vi "找螺丝刀方向-两头.vi"(8 "螺丝刀重心":cluster{"X":sgl, "Y":sgl} {"Y" format="%.2f"; "X" format="%.2f"}, 9 "Fitted Circle":T8, 11 "Img in":T5) -> (0 "螺丝刀中心":cluster{"X":sgl, "Y":sgl}, 1 "角度 2":dbl, 2 "铆点数量":i32, 3 "Image Out":T5, 4 "螺丝刀宽度":dbl)   [LabVIEW 2014]
uses:
  <vilib>/vision/Measure.llb/Edge Options.ctl
  <vilib>/vision/Measure.llb/Edge Polarity.ctl
  <vilib>/vision/Image Controls.llb/IMAQ Image.ctl
  <vilib>/vision/NI_Vision_Development_Module.lvlib
panel:
  out "角度 3":dbl
  out "Bisecting Line":T1 {"Point 2"."Y" format="%.2f"; "Point 2"."X" format="%.2f"; "Point 1"."Y" format="%.2f"; "Point 1"."X" format="%.2f"}
  in  "Options2":T4={"Search Direction"=1, "Edge Options"={"Edge Polarity"=1, "Kernel Size"=9, "Width"=3, "Minimum Edge Strength"=20.0, "Interpolation Type"=enum."Bilinear Fixed", "Data Processing Method"=enum."Average"}, "Show Search Area"=TRUE, "Show Search Lines"=FALSE, "Show Edges Found"=FALSE, "Show Result"=TRUE, "Search Area Color"=65280, "Search Lines Color"=255, "Edge Locations Color"=16776960, "Result Color"=16711680, "Overlay Group Name"=""} {"Edge Options"."Edge Polarity" items=["All Edges", "Rising Edges", "Falling Edges"]; "Edge Options"."Minimum Edge Strength" format="%.2f"; "Edge Options"."Width" step=2; "Edge Options"."Kernel Size" step=2; "Search Direction" items=["Left to Right", "Right to Left", "Top to Bottom", "Bottom to Top"]}
  in  "Options 2":T4={"Search Direction"=0, "Edge Options"={"Edge Polarity"=1, "Kernel Size"=9, "Width"=3, "Minimum Edge Strength"=20.0, "Interpolation Type"=enum."Bilinear Fixed", "Data Processing Method"=enum."Average"}, "Show Search Area"=TRUE, "Show Search Lines"=FALSE, "Show Edges Found"=FALSE, "Show Result"=TRUE, "Search Area Color"=65280, "Search Lines Color"=255, "Edge Locations Color"=16776960, "Result Color"=16711680, "Overlay Group Name"=""} {"Edge Options"."Edge Polarity" items=["All Edges", "Rising Edges", "Falling Edges"]; "Edge Options"."Minimum Edge Strength" format="%.2f"; "Edge Options"."Width" step=2; "Edge Options"."Kernel Size" step=2; "Search Direction" items=["Left to Right", "Right to Left", "Top to Bottom", "Bottom to Top"]}
  out "角度":dbl
  in  "Rectangle":T6 {"Rotation" min=-90.0 max=90.0 step=1.0 format="%.2f"; "Left" scale=0.0..1024.0; "Right" scale=0.0..1024.0}
  out "ROI out":T7={"Global Rectangle"=[921, 750, 1411, 1165], "Contours"=[{"ID"=enum."External", "Type"=12, "Coordinates"=[954, 797, 1378, 1118, 345974]}]} {"Contours"."Type" items=["No Selection", "Point", "Line", "Rectangle", "Oval", "Polygon", "Freehand Region", "Annulus", "Unused2", "Unused3", "Broken Line", "Freehand Line", "Rotated Rectangle"]}
  out "ROI中心":cluster{"X":dbl, "Y":dbl}
  out "存储缺口位置 2":cluster{"X":sgl, "Y":sgl}[](array[cluster])
  out "数组":i32[](array[numeric])
  out "i":i32
  out "存储当前铆点的默认位置":cluster{"X":sgl, "Y":sgl}[](array[cluster])
  out "存储缺口位置":cluster{"X":sgl, "Y":sgl}[](array[cluster])
  out "圆心到边距离 2":sgl[][](graph)
  out "输出数组 2":sgl[](array[numeric])
  in  "Options":T2={"Edge Polarity"=2, "Kernel Size"=5, "Width"=7, "Minimum Edge Strength"=20.0, "Interpolation Type"=enum."Bilinear Fixed", "Data Processing Method"=enum."Average"} {"Edge Polarity" items=["All Edges", "Rising Edges", "Falling Edges"]; "Minimum Edge Strength" format="%.2f"; "Width" step=2; "Kernel Size" step=2}
types:
  T1 = cluster{"Point 1":cluster{"X":sgl, "Y":sgl}, "Point 2":cluster{"X":sgl, "Y":sgl}}
  T2 = typedef "Edge Options.ctl" = cluster{"Edge Polarity":T3, "Kernel Size":u32, "Width":u32, "Minimum Edge Strength":sgl, "Interpolation Type":enum32{"Zero Order", "Bilinear", "Quadratic", "Cubic", "Bilinear Fixed"}, "Data Processing Method":enum32{"Average", "Median"}}
  T3 = typedef "Edge Polarity.ctl" = u32
  T4 = cluster{"Search Direction":u32, "Edge Options":T2, "Show Search Area":bool, "Show Search Lines":bool, "Show Edges Found":bool, "Show Result":bool, "Search Area Color":u32, "Search Lines Color":u32, "Edge Locations Color":u32, "Result Color":u32, "Overlay Group Name":string}
  T5 = typedef "IMAQ Image.ctl" = refnum<image>
  T6 = typedef "IMAQ Rectangle" = cluster{"Left":i32, "Top":i32, "Right":i32, "Bottom":i32, "Rotation":dbl}
  T7 = cluster{"Global Rectangle":i32[], "Contours":cluster{"ID":enum32{"External", "Internal"}, "Type":u32, "Coordinates":i32[]}[]}
  T8 = cluster{"Center (Pixels)":cluster{"X":sgl, "Y":sgl}, "Radius (Pixels)":dbl, "Center (Real-World)":cluster{"X":sgl, "Y":sgl}, "Radius (Real-World)":dbl, "Roundness (Real-World)":dbl, "Average Strength":dbl, "Average SNR (dB)":dbl}
  T9 = enum16{"Get First Edge", "Get First + Last Edge", "Get All Edges", "Get Best Edge"}
  T10 = typedef "ROI Descriptor" = cluster{"Global Rectangle":i32[], "Contours":cluster{"ID":enum32{"External", "Internal"}, "Type":u32, "Coordinates":i32[]}[]}
  T11 = typedef "Edge New.ctl" = cluster{"Location (Pixel)":cluster{"X":sgl, "Y":sgl}, "Location (Real-World)":cluster{"X":sgl, "Y":sgl}, "Distance (Pixel)":dbl, "Distance (Real-World)":dbl, "Strength":dbl, "Noise":dbl, "Rising?":bool}
  T12 = cluster{"存储缺口位置[0]":cluster{"X":sgl, "Y":sgl}, "存储缺口位置[1]":cluster{"X":sgl, "Y":sgl}}
  T13 = cluster{"Point1 (Pixels)":cluster{"X":sgl, "Y":sgl}, "Point2 (Pixels)":cluster{"X":sgl, "Y":sgl}, "Point1 (Real-World)":cluster{"X":sgl, "Y":sgl}, "Point2 (Real-World)":cluster{"X":sgl, "Y":sgl}, "Angle (Pixel)":dbl, "Angle (Real-World)":dbl, "Score":dbl, "Straightness":dbl, "Average SNR (db)":dbl, "Calibration Valid":bool}[]
  T14 = cluster{"Point1 (Pixels)":cluster{"X":sgl, "Y":sgl}, "Point2 (Pixels)":cluster{"X":sgl, "Y":sgl}, "Point1 (Real-World)":cluster{"X":sgl, "Y":sgl}, "Point2 (Real-World)":cluster{"X":sgl, "Y":sgl}, "Angle (Pixel)":dbl, "Angle (Real-World)":dbl, "Score":dbl, "Straightness":dbl, "Average SNR (db)":dbl, "Calibration Valid":bool}
  T15 = cluster{"Point1 (Pixels)":cluster{"X":sgl, "Y":sgl}, "Point2 (Pixels)":cluster{"X":sgl, "Y":sgl}}
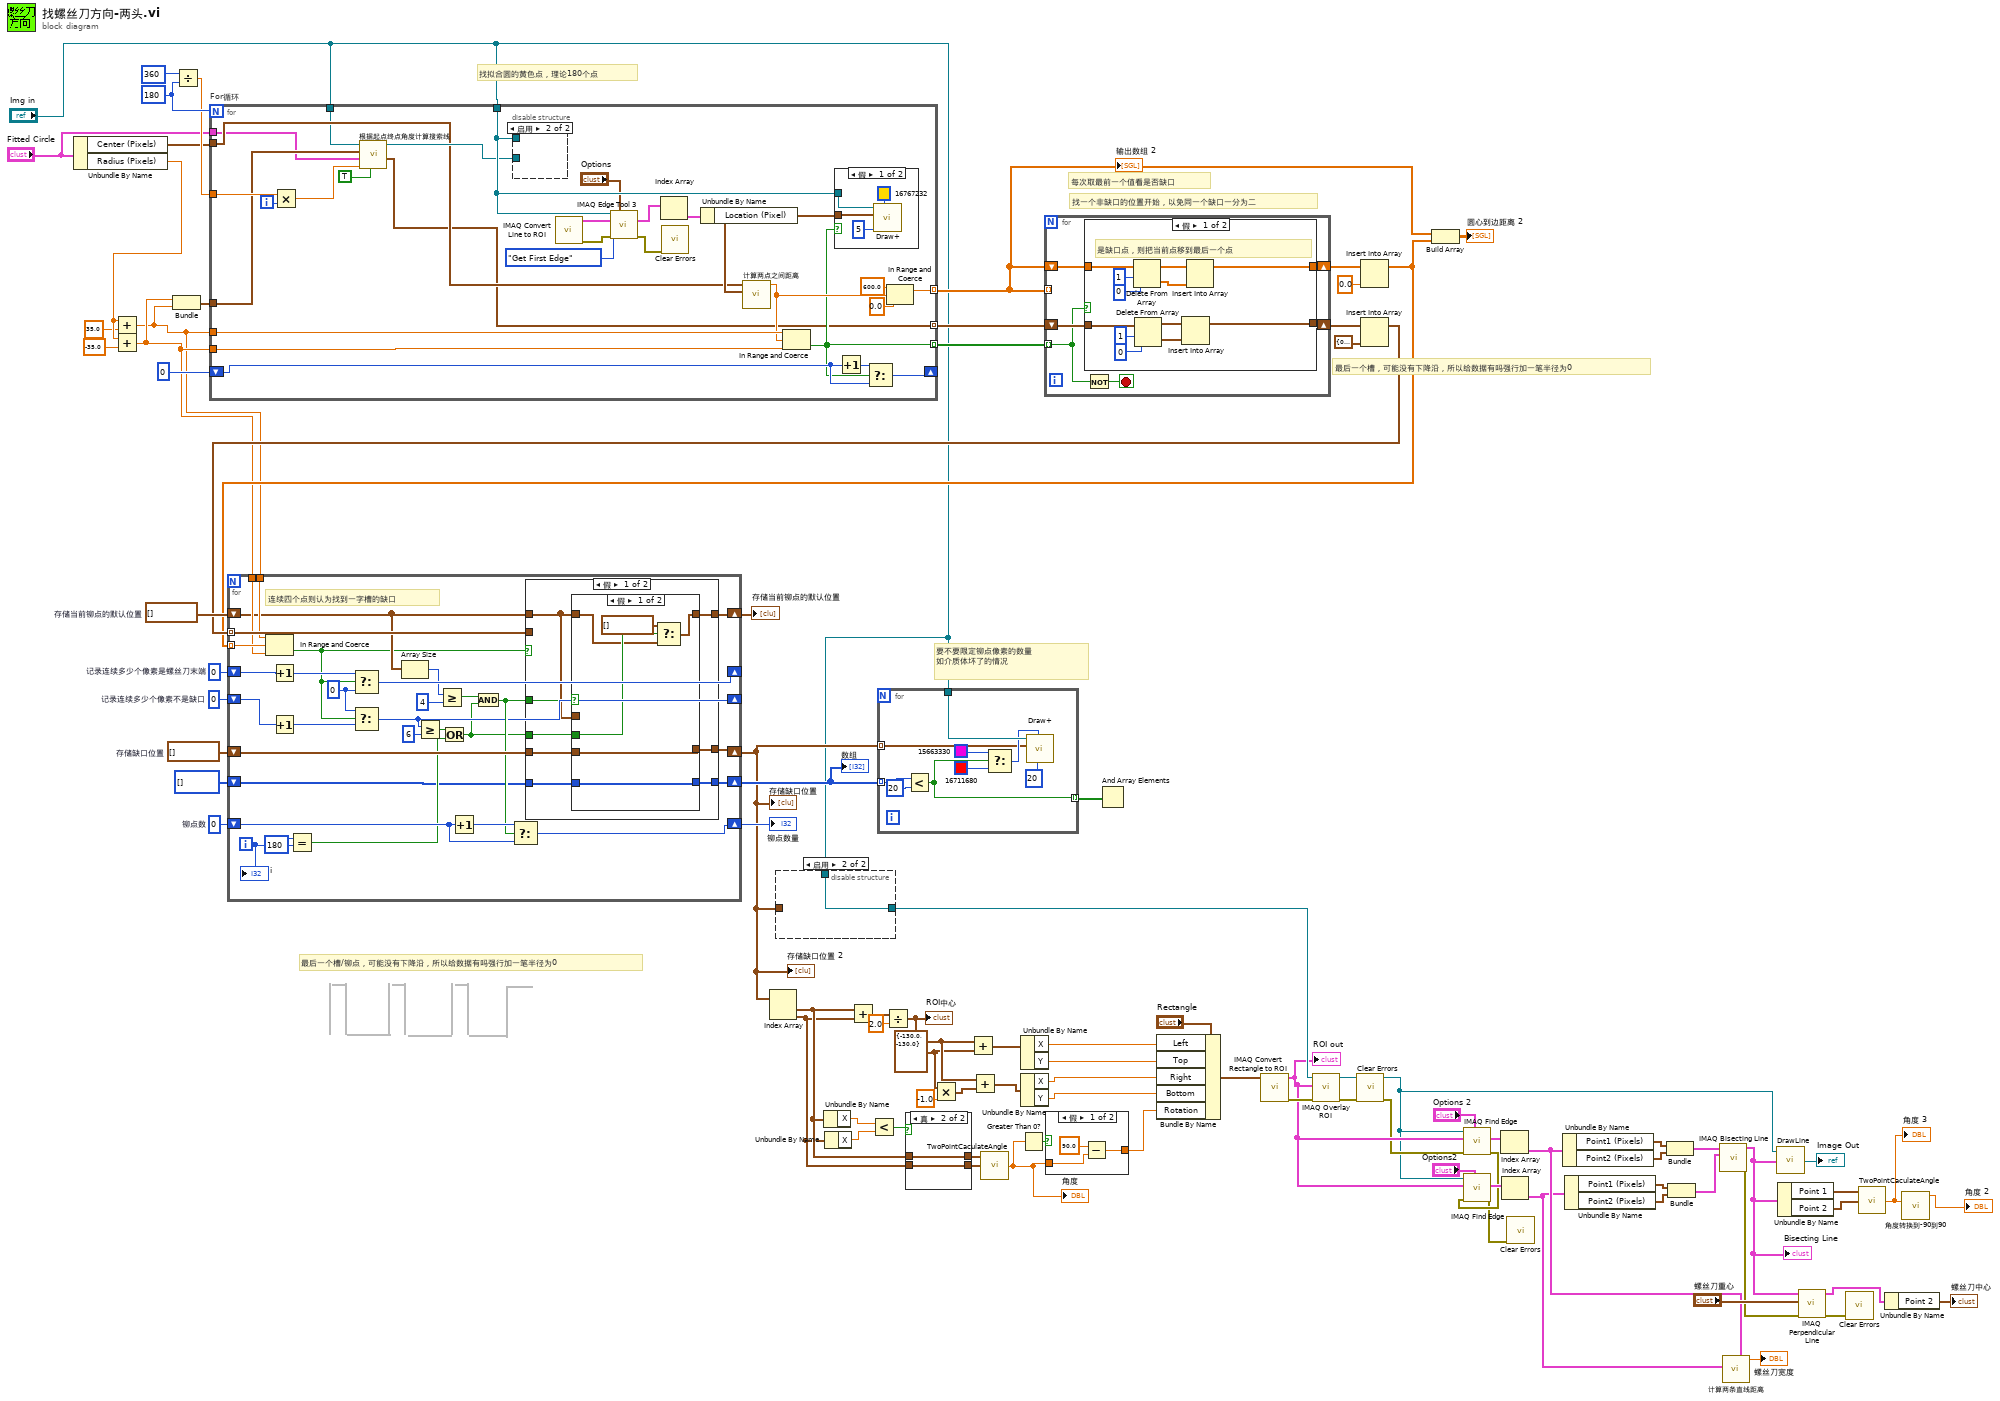
[diagram p0: block diagram]
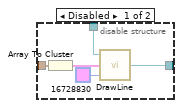
[diagram p2: hidden frame]
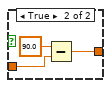
[diagram p3: hidden frame]
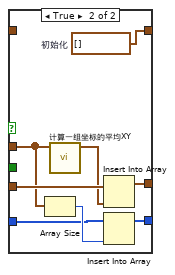
[diagram p6: hidden frame]
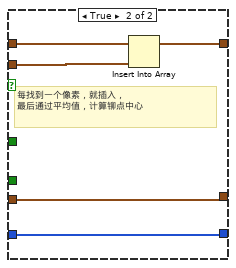
[diagram p7: hidden frame]
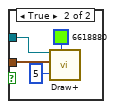
[diagram p8: hidden frame]
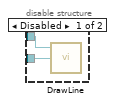
[diagram p9: hidden frame]
diagram:
  w57 = cluster{"X":dbl, "Y":dbl} {"X"=-130.0, "Y"=-130.0} ("y")
  w68 = 0  # 记录连续多少个像素不是缺口
  w84 = cluster{"X":sgl, "Y":sgl}[] []  # 存储缺口位置
  w85 = cluster{"X":sgl, "Y":sgl}[] []  # 存储当前铆点的默认位置
  w86 = 0  # 记录连续多少个像素是螺丝刀末端
  w87 = 0  # 铆点数
  w90 = 180
  # "要不要限定铆点像素的数量\n如介质体坏了的情况"
  # "最后一个槽，可能没有下降沿，所以给数据有吗强行加一笔半径为0"
  # "每次取最前一个值看是否缺口"
  # "最后一个槽/铆点，可能没有下降沿，所以给数据有吗强行加一笔半径为0"
  # "找拟合圆的黄色点，理论180个点"
  # "找一个非缺口的位置开始，以免同一个缺口一分为二"
  n1 = Unbundle By Name("Fitted Circle") -> ("Center (Pixels)"=w82:cluster{"X":sgl, "Y":sgl}, "Radius (Pixels)"=w72:dbl)
  n2 = Add(x=w72, y=35.0) -> (x+y=w3:dbl)
  n3 = Add(x=w72, y=-35.0) -> (x+y=w4:dbl)
  n4 = Bundle(w4, w3) -> (w2:cluster{dbl, dbl})  [unwired: 1 in]
  n5 = Divide(x=360, y=w90) -> (x/y=w89:dbl)
  n6 = for "For循环" {
    N: w90 -> [_]
    tunnel: w82 -> [w97]
    tunnel: "Img in" -> [w115]
    tunnel: w89 -> [w113]
    tunnel: [w106] -> w75 mode=indexing
    tunnel: [w91] -> w80 mode=indexing
    tunnel: w3 -> [w105]
    tunnel: w4 -> [w99]
    shift-right: [w103] -> _
    shift-left: 0 -> [w102]
    tunnel: [w96] -> w69 mode=indexing
    tunnel: "Img in" -> [w94]
    tunnel: w2 -> [w93]
    tunnel: "Fitted Circle" -> [w92]
    i -> [w119]
    n7 = Multiply(x=w113, y=w119) -> (x*y=w98:dbl)
    n8 = call "根据起点终点角度计算搜索线.vi"("从内外外搜索"=TRUE, "角度"=w98, "Fitted Circle"=w92, "内径外径"=w93, "Img in"=w94) -> ("找不到边界时默认点"=w91:cluster{dbl, dbl}, "Img out"=w100:T5)  [unwired: 4 in, 1 out]
    n9 = disable-structure shown="启用" {
      disable-tunnel: w100 -> [w129 _]
      disable-tunnel: w115 -> [w128 _]
      frame Disabled {
        n10 = call "DrawLine.vi"("Edge Points"=w129, "img in"=w128) -> ()  [unwired: 1 in, 1 out]
      }
      frame Enabled {
      }
    }
    n11 = call "IMAQ Convert Line to ROI"() -> ("error out"=w117:errorcluster, "ROI Descriptor"=w118:T10)  [unwired: 9 in]
    n12 = call "IMAQ Edge Tool 3"("Image"=w115, "Edge Options"="Options", "ROI Descriptor"=w118, "Process"=T9."Get First Edge", "error in (no error)"=w117) -> ("Edge Information"=w109:T11[], "error out"=w114:errorcluster)  [unwired: 6 in, 3 out]
    n13 = Index Array(array=w109) -> (element=w116:T11)  [unwired: 1 in]
    n14 = call <vilib>:"Clear Errors.vi"("error in (no error)"=w114) -> ()  [unwired: 5 in, 2 out]
    n15 = Unbundle By Name(w116) -> ("Location (Pixel)"=w110:cluster{"X":sgl, "Y":sgl})
    n16 = call "计算两点之间距离.vi"("Location (Pixel)"=w110, "Center (Pixels)"=w97) -> ("两点之间距离"=w101:sgl)  [unwired: 9 in]
    n17 = In Range and Coerce(upper limit=w105, x=w101, lower limit=w99) -> (In Range?=w96:bool)  [unwired: 1 out]
    n18 = case shown="假" w96 {
      tunnel: w115 -> [w122 w127]
      tunnel: w110 -> [w121 w126]
      frame False {
        n19 = call "Draw+.vi"("Width"=5, "Color"=u32 16767232, "input cluster"=w121, "Image In"=w122) -> ()  [unwired: 2 in, 1 out]
      }
      frame True {
        n20 = call "Draw+.vi"("Width"=5, "Color"=u32 6618880, "input cluster"=w126, "Image In"=w127) -> ()  [unwired: 2 in, 1 out]
      }
    }
    n21 = Increment(x=w102) -> (x+1=w104:i32)
    n22 = Select(t=w104, s=w96, f=w102) -> (s? t:f=w103:i32)
    n23 = In Range and Coerce(upper limit=sgl 600.0 ("上限"), x=w101, lower limit=sgl 0.0 ("下限")) -> (coerced(x)=w106:sgl)  [unwired: 1 out]
  }
  "输出数组 2" <- w75
  n24 = Multiply(x=w57, y=-1.0) -> (x*y=w58:cluster{"X":dbl, "Y":dbl})
  n25 = for {
    tunnel: w75 -> [_] mode=indexing
    shift-right: [w135] -> w77
    shift-left: w80 -> [w132]
    shift-right: [w134] -> w78
    shift-left: w75 -> [w131]
    tunnel: w69 -> [w130] mode=indexing
    stop <- w133 stop-if-true
    n26 = case shown="假" w130 {
      tunnel: w132 -> [w147 w148]
      tunnel: [w146 w148] -> w135
      tunnel: w131 -> [w143 w149]
      tunnel: [w142 w149] -> w134
      frame False {
        # "是缺口点，则把当前点移到最后一个点"
        n27 = Delete From Array(array=w143, length=1 ("长度"), index=0 ("索引")) -> (deleted portion=w136:sgl[], array with subset deleted=w145:sgl[])
        n28 = Delete From Array(array=w147, length=1 ("长度"), index=0 ("索引")) -> (deleted portion=w137:cluster{dbl, dbl}[], array with subset deleted=w140:cluster{dbl, dbl}[])
        n29 = Insert Into Array ("数组插入")(array=w140, new element=w137) -> (w146:cluster{dbl, dbl}[])  [unwired: 1 in]
        n30 = Insert Into Array ("数组插入")(array=w145, new element=w136) -> (w142:sgl[])  [unwired: 1 in]
      }
      frame True {
      }
    }
    n31 = Not(x=w130) -> (.not. x?=w133:bool)
  }
  n32 = Insert Into Array(array=w78, new element=sgl 0.0 ("新元素/子数组")) -> (w74:sgl[])  [unwired: 1 in]
  n33 = Insert Into Array(array=w77, new element=cluster{dbl, dbl} {0.0, 0.0} ("新元素/子数组")) -> (w76:cluster{dbl, dbl}[])  [unwired: 1 in]
  n34 = for {
    tunnel: w74 -> [w169] mode=indexing
    shift-right: [w179] -> w66
    shift-left: w87 -> [w178]
    shift-right: [w164] -> _
    shift-left: w86 -> [w166]
    tunnel: w76 -> [w177] mode=indexing
    shift-right: [w176] -> w67
    shift-left: w85 -> [w157]
    shift-right: [w174] -> w62
    shift-left: w84 -> [w175]
    tunnel: w3 -> [w168]
    tunnel: w4 -> [w167]
    shift-right: [w154] -> _
    shift-left: w68 -> [w163]
    shift-right: [w153] -> w64
    shift-left: i32[] [] -> [w152]
    i -> [w170]
    w161 = 0 ("f")
    # "连续四个点则认为找到一字槽的缺口"
    n35 = In Range and Coerce(upper limit=w168, x=w169, lower limit=w167) -> (In Range?=w150:bool)  [unwired: 1 out]
    n36 = Increment(x=w166) -> (x+1=w165:i32)
    n37 = Increment(x=w163) -> (x+1=w162:i32)
    n38 = Equal?(x=w170, y=180) -> (x = y?=w171:bool)
    n39 = Select(t=w165, s=w150, f=w161) -> (s? t:f=w164:i32)
    n40 = Select(t=w161, s=w150, f=w162) -> (s? t:f=w154:i32)
    n41 = Array Size(array=w157) -> (size(s)=w156:i32)
    n42 = Greater Or Equal?(x=w154, y=6) -> (x >= y?=w159:bool)
    n43 = Greater Or Equal?(x=w156, y=4) -> (x >= y?=w158:bool)
    n44 = Or(x=w159, y=w171) -> (x .or. y?=w151:bool)
    n45 = Increment(x=w178) -> (x+1=w180:i32)
    n46 = And(x=w158, y=w151) -> (x .and. y?=w173:bool)
    n47 = Select(t=w180, s=w173, f=w178) -> (s? t:f=w179:i32)
    n48 = case shown="假" w150 {
      tunnel: w157 -> [w184 w207]
      tunnel: w177 -> [_ w206]
      tunnel: [w185 w205] -> w176
      tunnel: w175 -> [w188 w204]
      tunnel: w173 -> [w186 _]
      tunnel: [w187 w204] -> w174
      tunnel: [w183 w203] -> w153
      tunnel: w152 -> [w182 w203]
      tunnel: w151 -> [w181 _]
      frame False {
        n49 = case shown="假" w186 {
          tunnel: w184 -> [_ w198]
          tunnel: w188 -> [w194 w202]
          tunnel: [w194 w200] -> w187
          tunnel: [w190 w199] -> w185
          tunnel: w184 -> [w191 _]
          tunnel: [w193 w196] -> w183
          tunnel: w182 -> [w193 w195]
          tunnel: w181 -> [w192 _]
          frame False {
            n50 = Select(t=cluster{"X":sgl, "Y":sgl}[] [], s=w192, f=w191) -> (s? t:f=w190:cluster{"X":sgl, "Y":sgl}[])
          }
          frame True {
            w199 = cluster{"X":sgl, "Y":sgl}[] []  # 初始化
            n51 = Array Size(array=w198) -> (size(s)=w197:i32)
            n52 = call "计算一组坐标的平均XY.vi"("存储当前铆点的默认位置"=w198) -> ("簇"=w201:cluster{"mean":dbl, "mean":dbl})  [unwired: 9 in, 1 out]
            n53 = Insert Into Array(array=w202, new element=w201) -> (w200:cluster{"X":sgl, "Y":sgl}[])  [unwired: 1 in]
            n54 = Insert Into Array(array=w195, new element=w197) -> (w196:i32[])  [unwired: 1 in]
          }
        }
      }
      frame True {
        # "每找到一个像素，就插入，\n最后通过平均值，计算铆点中心"
        n55 = Insert Into Array(array=w207, new element=w206) -> (w205:cluster{"X":sgl, "Y":sgl}[])  [unwired: 1 in]
      }
    }
    "i" <- w170
  }
  "铆点数量" <- w66
  "存储缺口位置" <- w62
  "存储当前铆点的默认位置" <- w67
  "数组" <- w64
  "存储缺口位置 2" <- w62
  n56 = Index Array(array=w62) -> (element #1=w41:cluster{"X":sgl, "Y":sgl}, element #2=w40:cluster{"X":sgl, "Y":sgl})  [unwired: 2 in]
  n57 = disable-structure shown="启用" {
    disable-tunnel: "Img in" -> [w211 w213]
    disable-tunnel: w62 -> [w210 _]
    disable-tunnel: [w209 w213] -> w45
    frame Disabled {
      n58 = Array To Cluster(array=w210) -> (cluster=w212:T12)
      n59 = call "DrawLine.vi"("Color"=u32 16728830, "Edge Points"=w212, "img in"=w211) -> ("Image Out"=w209:T5)
    }
    frame Enabled {
    }
  }
  n60 = Unbundle By Name(w41) -> ("X"=w44:sgl)
  n61 = Unbundle By Name(w40) -> ("X"=w43:sgl)
  n62 = Add(x=w41, y=w40) -> (x+y=w61:cluster{"X":sgl, "Y":sgl})
  n63 = Less?(x=w44, y=w43) -> (x < y?=w42:bool)
  n64 = for {
    tunnel: "Img in" -> [w222]
    tunnel: w62 -> [w217] mode=indexing
    tunnel: w64 -> [w216] mode=indexing
    tunnel: [w214] -> w63 mode=indexing
    n65 = Less?(x=w216, y=20) -> (x < y?=w214:bool)
    n66 = Select(t=u32 15663330 ("Color"), s=w214, f=u32 16711680 ("Color")) -> (s? t:f=w218:u32)
    n67 = call "Draw+.vi"("Width"=20, "Color"=w218, "input cluster"=w217, "Image In"=w222) -> ()  [unwired: 2 in, 1 out]
  }
  n68 = Divide(x=w61, y=2.0) -> (x/y=w59:cluster{"X":dbl, "Y":dbl})
  "ROI中心" <- w59
  n69 = case shown="真" w42 {
    tunnel: w41 -> [w223 w226]
    tunnel: w40 -> [w224 w225]
    tunnel: [w224 w226] -> w39
    tunnel: [w223 w225] -> w38
    frame False {
    }
    frame True {
    }
  }
  n70 = Add(x=w59, y=w57) -> (x+y=w55:cluster{"X":dbl, "Y":dbl})
  n71 = Add(x=w59, y=w58) -> (x+y=w54:cluster{"X":dbl, "Y":dbl})
  n72 = call "TwoPointCaculateAngle.vi"("Point2"=w38, "Point1"=w39) -> ("角度"=w35:dbl)  [unwired: 1 in]
  "角度" <- w35
  n73 = Greater Than 0?(x=w35) -> (x > 0?=w36:bool)
  n74 = Unbundle By Name(w55) -> ("X"=w52:dbl, "Y"=w51:dbl)
  n75 = Unbundle By Name(w54) -> ("X"=w50:dbl, "Y"=w49:dbl)
  n76 = case shown="假" w36 {
    tunnel: [w227 w231] -> w37
    tunnel: w35 -> [w228 w230]
    frame False {
      n77 = Subtract(x=90.0, y=w228) -> (x-y=w227:dbl)
    }
    frame True {
      n78 = Subtract(x=90.0, y=w230) -> (x-y=w231:dbl)
    }
  }
  n79 = And Array Elements(Boolean array=w63) -> ()  [unwired: 1 out]
  n80 = Bundle By Name(cluster="Rectangle", "Left"=w52, "Top"=w51, "Right"=w50, "Bottom"=w49, "Rotation"=w37) -> (w48:T6)
  n81 = call "IMAQ Convert Rectangle to ROI"("Rectangle"=w48) -> ("error out"=w47:errorcluster, "ROI Descriptor"=w23:T10)  [unwired: 8 in]
  "ROI out" <- w23
  n82 = call "IMAQ Overlay ROI"("error in (no error)"=w47, "ROI Descriptor"=w23, "Image"=w45) -> ("error out"=w46:errorcluster, "Image Out"=w19:T5)  [unwired: 7 in]
  n83 = call <vilib>:"Clear Errors.vi"("error in (no error)"=w46) -> ("error out"=w22:errorcluster)  [unwired: 5 in, 1 out]
  n84 = Build Array(w75, w74) -> (→"圆心到边距离 2":sgl[][])
  n85 = call "IMAQ Find Edge"("Options"="Options 2", "error in (no error)"=w22, "ROI Descriptor"=w23, "Image"=w19) -> ("error out"=w21:errorcluster, "Straight Edges"=w32:T13)  [unwired: 4 in, 2 out]
  n86 = call "IMAQ Find Edge"("Options"="Options2", "error in (no error)"=w21, "ROI Descriptor"=w23, "Image"=w19) -> ("error out"=w20:errorcluster, "Straight Edges"=w27:T13)  [unwired: 4 in, 2 out]
  n87 = Index Array(array=w32) -> (element=w7:T14)  [unwired: 1 in]
  n88 = Index Array(array=w27) -> (element=w6:T14)  [unwired: 1 in]
  n89 = call <vilib>:"Clear Errors.vi"("error in (no error)"=w20) -> ()  [unwired: 5 in, 2 out]
  n90 = Unbundle By Name(w7) -> ("Point1 (Pixels)"=w31:cluster{"X":sgl, "Y":sgl}, "Point2 (Pixels)"=w30:cluster{"X":sgl, "Y":sgl})
  n91 = Unbundle By Name(w6) -> ("Point1 (Pixels)"=w28:cluster{"X":sgl, "Y":sgl}, "Point2 (Pixels)"=w29:cluster{"X":sgl, "Y":sgl})
  n92 = Bundle("Point1 (Pixels)"=w31, "Point2 (Pixels)"=w30) -> (w8:T15)  [unwired: 1 in]
  n93 = Bundle("Point1 (Pixels)"=w28, "Point2 (Pixels)"=w29) -> (w26:T15)  [unwired: 1 in]
  n94 = call "IMAQ Bisecting Line"("Line 2"=w26, "Line 1"=w8) -> ("error out"=w12:errorcluster, "Bisecting Line"=w17:T1)  [unwired: 8 in]
  "Bisecting Line" <- w17
  n95 = call "计算两条直线距离.vi"("Straight Edge (下直线)"=w6, "Straight Edge (上直线)"=w7) -> ("Distance"=→"螺丝刀宽度":dbl)  [unwired: 9 in]
  n96 = call "DrawLine.vi"("Edge Points"=w17, "img in"=w19) -> ("Image Out"=→"Image Out":T5)  [unwired: 1 in]
  n97 = Unbundle By Name(w17) -> ("Point 1"=w25:cluster{"X":sgl, "Y":sgl}, "Point 2"=w24:cluster{"X":sgl, "Y":sgl})
  n98 = call "IMAQ Perpendicular Line"("error in (no error)"=w12, "Point"="螺丝刀重心", "Line"=w17) -> ("error out"=w15:errorcluster, "Perpendicular Line"=w14:T1)  [unwired: 6 in, 1 out]
  n99 = call <vilib>:"Clear Errors.vi"("error in (no error)"=w15) -> ()  [unwired: 5 in, 2 out]
  n100 = call "TwoPointCaculateAngle.vi"("Point2"=w24, "Point1"=w25) -> ("角度"=w11:dbl)  [unwired: 1 in]
  "角度 3" <- w11
  n101 = Unbundle By Name(w14) -> ("Point 2"=→"螺丝刀中心":cluster{"X":sgl, "Y":sgl})
  n102 = call "角度转换到-90到90.vi"("数值输入"=w11) -> ("数值输出"=→"角度 2":dbl)  [unwired: 10 in]
